vi "SDL_Image Test.vi"() -> ()   [LabVIEW 2014]
uses:
  Libraries/LibSDL2 Wrapper/Controls/Init Flags.ctl
  Libraries/LibSDL2 Wrapper/LibSDL2.lvlib
  Libraries/LibSDL2_Image Wrapper/LibSDL2_Image.lvlib
panel:
  out "Error":string
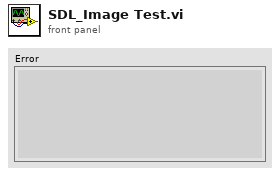
[diagram p1: front panel]
types:
  T1 = typedef "LibSDL2.lvlib/Init Flags.ctl" = u32
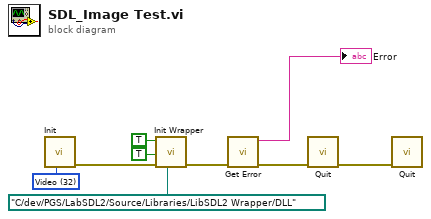
[diagram p0: block diagram]
diagram:
  w9 = T1 32 items=["Timer"=1, "Audio"=16, "Video"=32, "Joystick"=512, "Haptic"=4096, "Game Controller"=8192, "Events"=16384, "No Parachute"=1048576, "Everything"=17244689] ("Init Flags")
  n1 = call "Init.vi"("Flags"=w9) -> ("error out"=w5:errorcluster)  [unwired: 9 in, 1 out]
  n2 = call "Init Wrapper.vi"("DLL Directory"=path "C:/dev/PGS/LabSDL2/Source/Libraries/LibSDL2 Wrapper/DLL" ("Path"), "error in"=w5, "JPG (F)"=TRUE, "PNG (F)"=TRUE ("PNG")) -> ("error out"=w4:errorcluster)  [unwired: 6 in, 1 out]
  n3 = call "Get Error.vi"("error in"=w4) -> ("error out"=w3:errorcluster, "Error"=→"Error":string)  [unwired: 9 in]
  n4 = call "Quit.vi"("error in"=w3) -> ("error out"=w7:errorcluster)  [unwired: 10 in]
  n5 = call "Quit.vi"("error in"=w7) -> ()  [unwired: 10 in, 1 out]
